vi "Switch Configuration - Channel Array from Topology.vi"(8 "error in (no error)":errorcluster, 10 "Selected Mux Topology":string) -> (0 "error out":errorcluster, 2 "Channel Array Out":string[](array[string]))   [LabVIEW 2015, in "DMM-SWITCH-ScanList System Explorer.lvlib"]
doc: "Generate a Channel Array based on a specific Mux with a specific Topology"
uses:
  DMM-SWITCH-ScanList System Explorer.lvlib
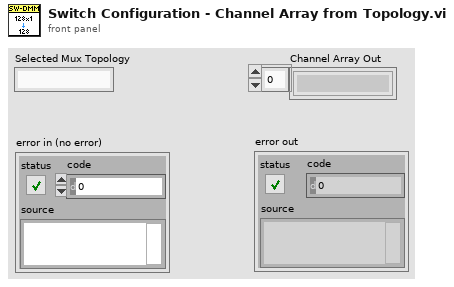
[diagram p1: front panel]
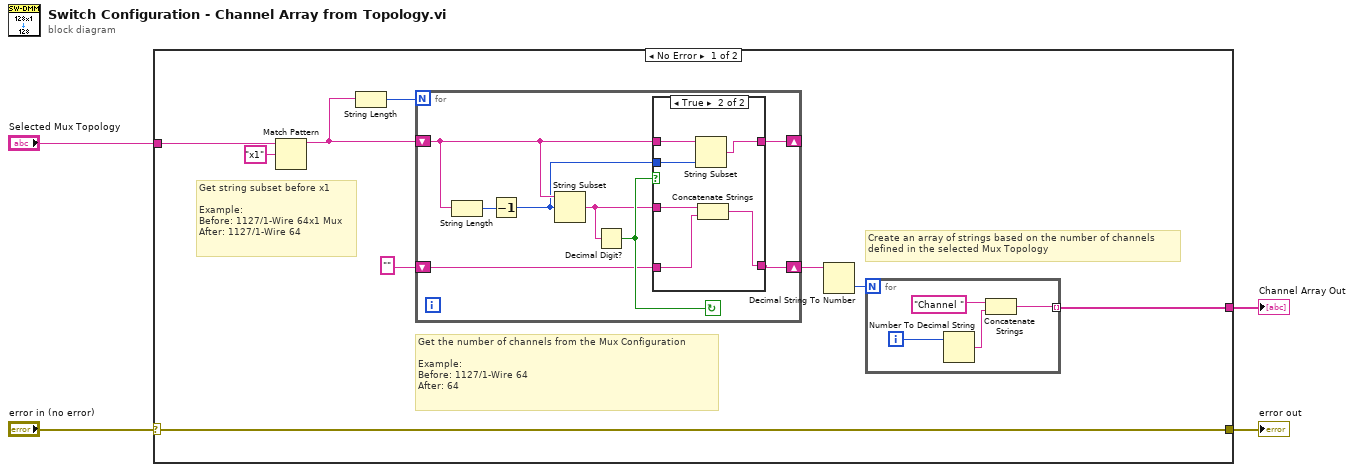
[diagram p0: block diagram]
diagram:
  n1 = case shown="No Error" "error in (no error)" {
    selector: "error in (no error)" -> [w5 w34]
    tunnel: "Selected Mux Topology" -> [w13 _]
    tunnel: [w6 _] -> w3
    tunnel: [w5 w34] -> w1
    frame No Error {
      # "Create an array of strings based on the number of channels\ndefined in the selected Mux Topology"
      # "Get the number of channels from the Mux Configuration\n\nExample:\nBefore: 1127/1-Wire 64 \nAfter: 64"
      # "Get string subset before x1\n\nExample:\nBefore: 1127/1-Wire 64x1 Mux\nAfter: 1127/1-Wire 64"
      n2 = Match Pattern(string=w13, regular expression="x1") -> (before substring=w10:string)  [unwired: 1 in, 3 out]
      n3 = String Length(string=w10) -> (length=w9:i32)
      n4 = for {
        N: w9 -> [_]
        shift-right: [w18] -> _
        shift-left: w10 -> [w20]
        shift-right: [w14] -> w7
        shift-left: "" -> [w16]
        stop <- w17 continue-if-true
        n5 = String Length(string=w20) -> (length=w21:i32)
        n6 = Decrement(x=w21) -> (x-1=w19:i32)
        n7 = String Subset(string=w20, offset (0)=w19) -> (substring=w15:string)  [unwired: 1 in]
        n8 = Decimal Digit?(1:w15) -> (0:w17:bool)
        n9 = case shown="True" w17 {
          tunnel: w20 -> [w23 w29]
          tunnel: w19 -> [_ w27]
          tunnel: [w23 w28] -> w18
          tunnel: w16 -> [w22 w24]
          tunnel: w15 -> [_ w25]
          tunnel: [w22 w26] -> w14
          frame False {
          }
          frame True {
            n10 = String Subset(string=w29, length (rest)=w27) -> (substring=w28:string)  [unwired: 1 in]
            n11 = Concatenate Strings(w25, w24) -> (w26:string)
          }
        }
      }
      n12 = Decimal String To Number(string=w7) -> (number=w12:i32)  [unwired: 2 in, 1 out]
      n13 = for {
        N: w12 -> [_]
        tunnel: [w30] -> w6 mode=indexing
        i -> [w31]
        n14 = Number To Decimal String(number=w31) -> (decimal integer string=w32:string)  [unwired: 1 in]
        n15 = Concatenate Strings("Channel ", w32) -> (w30:string)
      }
    }
    frame Error {
    }
  }
  "Channel Array Out" <- w3
  "error out" <- w1
